vi "Focus Move Absolute.vi"(8 "error in (no error)":errorcluster, 9 "Position":i32, 10 "Motor (0:n-1)":i32, 11 "ArduinoFocus in":refnum<class "ArduinoFocus.lvclass">) -> (0 "error out":errorcluster, 3 "ArduinoFocus out":refnum<class "ArduinoFocus.lvclass">)   [LabVIEW 2022 SP3, in "ArduinoFocus.lvclass"]
uses:
  ArduinoFocus.lvclass
  ArduinoFocus.lvclass/ArduinoFocus.ctl
  Focus Class/Focus Class.lvclass
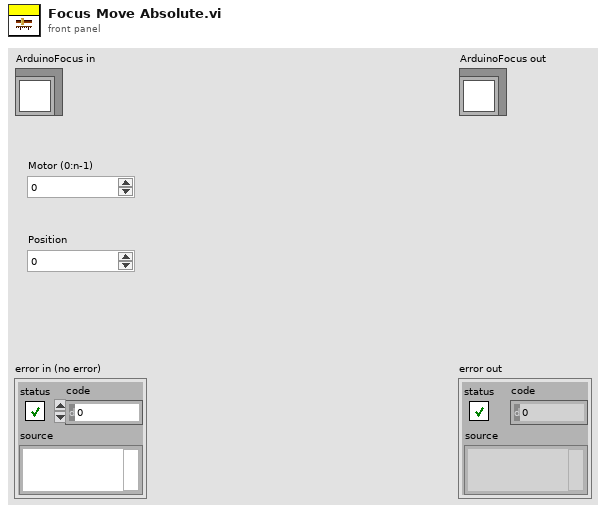
[diagram p1: front panel]
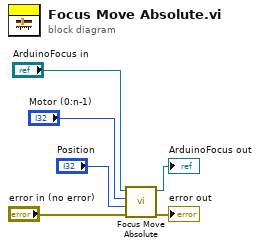
[diagram p0: block diagram]
diagram:
  n1 = call-parent "Focus Move Absolute.vi"("error in (no error)"="error in (no error)", "Position"="Position", "Motor (0:n-1)"="Motor (0:n-1)", "Focus Class in"="ArduinoFocus in") -> ("error out"=→"error out":errorcluster, "Focus Class out"=→"ArduinoFocus out":refnum<class "ArduinoFocus.lvclass">)  [unwired: 6 in]
